vi "Windows UI.vi"() -> ()   [LabVIEW 2014]
doc: "This is the primary Host VI."
panel:
  in  "IP Address":string="10.0.0.2"
  out "Display Battery State":bool
  out "Current Temperature":dbl(knob) scale=20.0..40.0
  out "Battery State":enum16{"Charged", "Running", "Low Batt"}(ring)
  out "Display RPM":bool
  out "Display Temperature":bool
  out "Display Voltage":bool
  out "Temperature Warning":bool
  out "Current RPM":dbl(knob) scale=0.0..1000.0
  in  "Stop Button":bool
  out "Error Out":errorcluster
  out "Current Voltage":dbl(knob) scale=0.0..4.0
  out "Variable History":cluster{dbl, dbl, dbl}(graph)
  # "NOTE: Update with your eval device IP address and select Edit>>Make Current Values Default before running"
  # "LCD Controls"
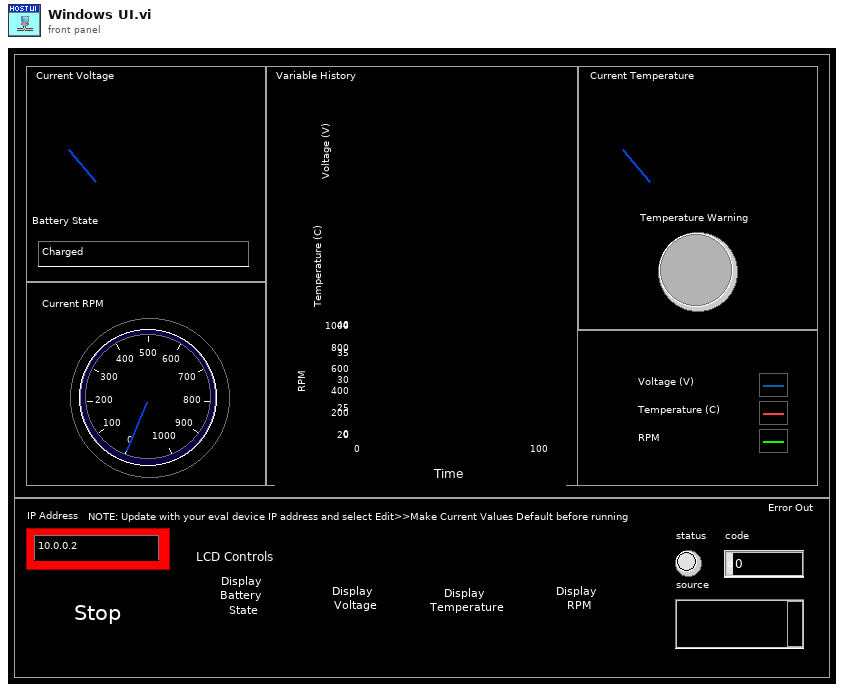
[diagram p1: front panel]
types:
  T1 = cluster{"Temperature Ref":refnum<k21>, "Temperature Warning Ref":refnum<k21>, "Voltage Ref":refnum<k21>, "Battery State Ref":refnum<k21>, "RPM Ref":refnum<k21>, "Display State Ref":refnum<k21>}
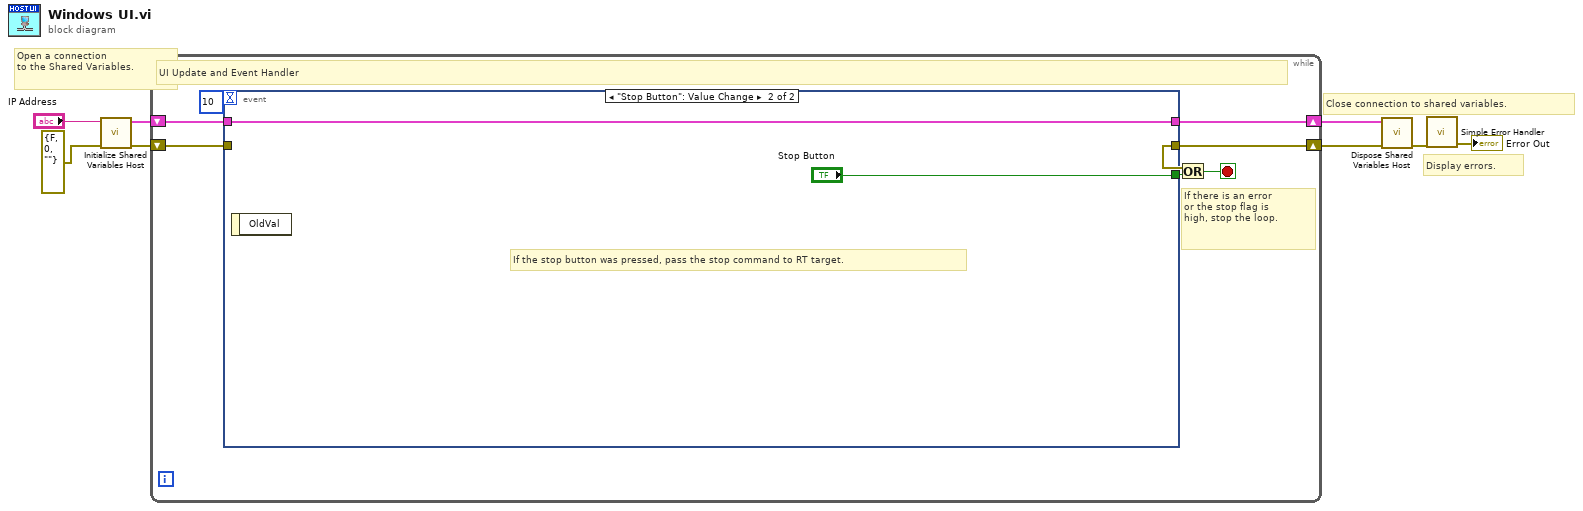
[diagram p0: block diagram]
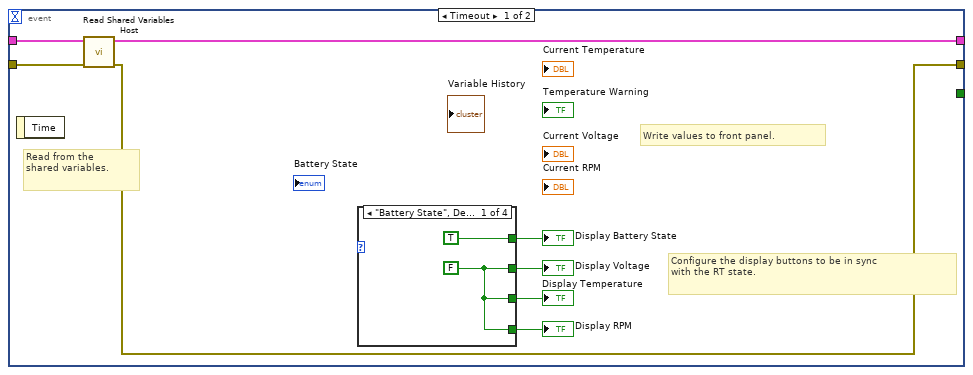
[diagram p2: hidden frame]
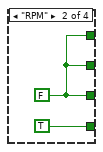
[diagram p3: hidden frame]
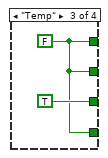
[diagram p4: hidden frame]
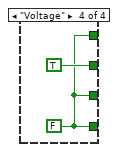
[diagram p5: hidden frame]
diagram:
  # "Close connection to shared variables."
  # "Display errors."
  # "Open a connection\nto the Shared Variables."
  n1 = call "Initialize Shared Variables Host.vi"("error in (no error)"=errorcluster {"status"=FALSE, "code"=0, "source"=""} ("error out"), "IP Address (No Slashes)"="IP Address") -> ("error out"=w7:errorcluster, "Shared Variable References"=w8:T1)  [unwired: 8 in]
  n2 = while {
    shift-right: [w10] -> w5
    shift-left: w7 -> [w15]
    shift-right: [w12] -> w6
    shift-left: w8 -> [w13]
    stop <- w11 stop-if-true
    # "UI Update and Event Handler"
    # "If there is an error\nor the stop flag is \nhigh, stop the loop."
    n3 = event shown="[1] \"Stop Button\": Value Change" {
      selector: _ -> [_ _]
      dyn-events: _ -> [_ _]
      timeout: 10 -> [_ _]
      tunnel: [w21 _] -> w10
      tunnel: w15 -> [w22 _]
      tunnel: w13 -> [w23 w33]
      tunnel: [w16 w33] -> w12
      tunnel: [_ "Stop Button"] -> w9
      event Timeout {
        # "Write values to front panel."
        # "Read from the\nshared variables."
        # "Configure the display buttons to be in sync\nwith the RT state."
        n4 = event-data() -> ()  [unwired: 1 in, 1 out]
        n5 = call "Read Shared Variables Host.vi"("error in (no error)"=w22, "Shared Variable References"=w23) -> ("error out"=w21:errorcluster, "Shared Variable References Out"=w16:T1)  [unwired: 7 in, 1 out]
        n6 = case shown="\"Battery State\", Default" {
          selector: _ -> [_ _ _ _]
          tunnel: [TRUE ("Display Battery State") w26 w28 w30] -> w20
          tunnel: [w24 w26 w28 TRUE ("Display Battery State")] -> w19
          tunnel: [w24 w26 TRUE ("Display Battery State") w30] -> w18
          tunnel: [w24 TRUE ("Display Battery State") w28 w30] -> w17
          frame "Battery State", Default {
            w24 = FALSE
          }
          frame "RPM" {
            w26 = FALSE
          }
          frame "Temp" {
            w28 = FALSE
          }
          frame "Voltage" {
            w30 = FALSE
          }
        }
        "Display Battery State" <- w20
        "Display Voltage" <- w19
        "Display Temperature" <- w18
        "Display RPM" <- w17
      }
      event "Stop Button": Value Change {
        # "If the stop button was pressed, pass the stop command to RT target."
        n7 = event-data() -> ()  [unwired: 1 in, 1 out]
      }
    }
    n8 = Or(x=w10, y=w9) -> (x .or. y?=w11:bool)
  }
  n9 = call "Dispose Shared Variables Host.vi"("error in (no error)"=w5, "Shared Variable References"=w6) -> ("error out"=w2:errorcluster)  [unwired: 9 in]
  n10 = call <vilib>:"Simple Error Handler.vi"("error in (no error)"=w2) -> ("error out"=→"Error Out":errorcluster)  [unwired: 4 in, 4 out]
